vi "To String (Boolean).vi"(7 "enable LabVIEW extensions? (T)":bool=TRUE, 8 "error in (no error)":errorcluster, 11 "JSON Value in":refnum<class "JSON Value.lvclass">) -> (0 "error out":errorcluster, 3 "String":string)   [LabVIEW 2016, in "JSON Value.lvclass"]
uses:
  JSON Value.lvclass
  JSON Value.lvclass/JSON Value.ctl
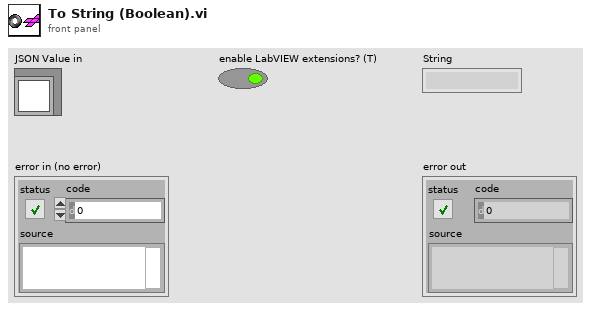
[diagram p1: front panel]
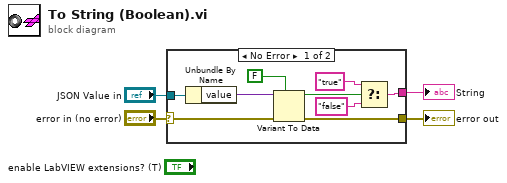
[diagram p0: block diagram]
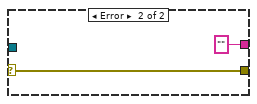
[diagram p2: hidden frame]
diagram:
  n1 = case shown="No Error" "error in (no error)" {
    selector: "error in (no error)" -> [w7 w14]
    tunnel: "JSON Value in" -> [w13 _]
    tunnel: [w9 "" ("f")] -> w3
    tunnel: [w6 w14] -> w1
    frame No Error {
      n2 = Unbundle By Name(w13) -> ("value"=w12:variant)
      n3 = Variant To Data(error in=w7, type=FALSE, Variant=w12) -> (data=w5:bool, error out=w6:errorcluster)
      n4 = Select(t="true" ("String"), s=w5, f="false") -> (s? t:f=w9:string)
    }
    frame Error {
    }
  }
  "String" <- w3
  "error out" <- w1
